vi "CleanHandler.init clean afg.vi"(0 "i ref in":refnum<vi>, 1 "CleanAfg":i32, 2 "amplitude [V]":dbl format="%.2f", 3 "ms timeout (100)":i32=100, 4 "frequency [Hz]":dbl format="%.2f", 5 "error in (no error)":errorcluster) -> (14 "i ref out":refnum<vi>, 17 "timed out":bool, 19 "error out":errorcluster)   [LabVIEW 2014, in "CleanHandler.lvlib"]
doc: "Sets the frequency [Hz] and amplitude [V] at the AFG with number CleanAFG. The numbering of the CleanAFGs starts with 0."
uses:
  CleanHandler.lvlib
  CS_Core/CSSystem/CoreDefs/CoreDefs.error_type.ctl
  CS_Core/CSSystem/CoreLib/CoreLib.double 2 byte array.vi
  CS_Core/CSSystem/CoreLib/CoreLib.lvlib
  CS_Core/BaseProcess/BaseProcess.lvlib
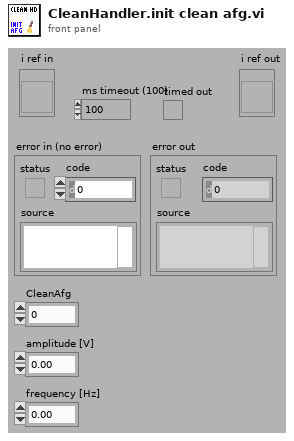
[diagram p1: front panel]
types:
  T1 = typedef "CoreDefs.error_type.ctl" = enum16{"no error", "can't load process", "can't unload process", "process does not exist", "can't install process", "can't remove process", "unknown function", "time out", "can't execute function", "duplicate queue name", "super not found", "caller queue invalid", "can't ping process", "unknown error", "VISA Error", "VISA timeout", "GPIB timeout", "GPIB error", "communication error", "data type mismatch", "can't read data from OPC server", "can't write data to OPC server", "OET error", "function not implemented", "process already exists", "invalid Shared Variable name", "error writing Shared Variable", "error reading Shared Variable", "invalid client name", "corrupt database", "unknown class", "call not authorized", "parameter out of range", "OET timeout: can't get data to modify", "invalid queue name", "requested operation incompatible with current state", "event undefined", "event disabled", "state undefined", "caller is not a friend", "EventBuilder: bad eventID", "EventBuilder: no DAQ devices", "a thread must not stop itself", "UNUSED ELEMENT4", "DiscArchiver: eventData incomplete", "DiscArchiver: eventData does not belong to run", "DiscArchiver: can't open file", "DiscArchiver: can't write to file", "DiscArchiver: available disc space low", "can't acquire semaphore", "error reading data from database", "notifier object is not existing", "can't register process", "can't unregister process", "illegal event type", "object disabled", "object already exists", "can't change state", "Instrument not found", "no connection to remote node", "invalid reference", "N/A", "UNUSED ELEMENT 1", "element not found", "illegal TCP/IP connection detected", "object does not exist", "invalid access ID", "unknown CS system", "invalid privilige", "unsupported data type", "unsupported server type", "IO server already exists", "Shared Variable already exists"}
  T2 = enum16{"simple", "synchronous", "asynchronous", "notification"}
  T3 = typedef "CoreDefs.rawDataType.ctl" = i8[]
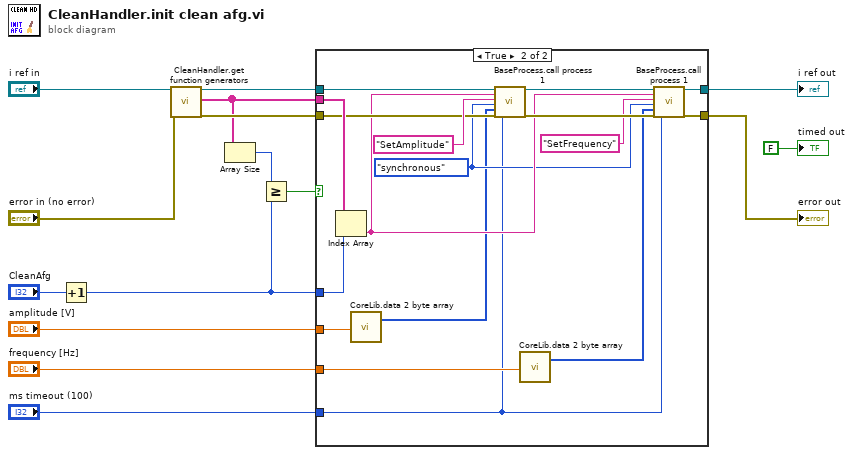
[diagram p0: block diagram]
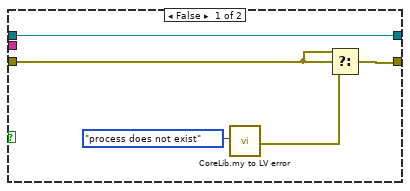
[diagram p2: hidden frame]
diagram:
  n1 = Increment(x="CleanAfg") -> (x+1=w5:i32)
  n2 = call "CleanHandler.get function generators.vi"("i ref in"="i ref in", "error in (no error)"="error in (no error)") -> ("i ref out"=w10:refnum<vi>, "function generators"=w6:string[], "error out"=w8:errorcluster)  [unwired: 14 in, 1 out]
  n3 = Array Size(array=w6) -> (size(s)=w12:i32)
  n4 = Greater Or Equal?(x=w12, y=w5) -> (x >= y?=w11:bool)
  n5 = case shown="True" w11 {
    tunnel: [w20 w31] -> w9
    tunnel: w10 -> [w20 w37]
    tunnel: w8 -> [w18 w33]
    tunnel: [w19 w30] -> w7
    tunnel: w6 -> [_ w36]
    tunnel: w5 -> [_ w35]
    tunnel: "amplitude [V]" -> [_ w32]
    tunnel: "frequency [Hz]" -> [_ w24]
    tunnel: "ms timeout (100)" -> [_ w23]
    frame False {
      n6 = call "CoreLib.my to LV error.vi"("ErrorTypes"=CoreDefs.error_type."process does not exist") -> ("myErrorCluster"=w17:errorcluster)  [unwired: 17 in, 1 out]
      n7 = Select(t=w18, s=w18, f=w17) -> (s? t:f=w19:errorcluster)
    }
    frame True {
      w25 = T2."synchronous" ("CallType")
      n8 = Index Array(array=w36, index=w35) -> (element=w27:string)
      n9 = call-poly "CoreLib.data 2 byte array.vi"("f64"=w32) -> ("byteArray out"=w21:T3)  [unwired: 18 in]
      n10 = call "BaseProcess.call process 1.vi"("i ref in"=w37, "Object"=w27, "Selector"="SetAmplitude", "CallType"=w25, "Data"=w21, "error in (no error)"=w33, "timeout (ms)"=w23) -> ("i ref out"=w29:refnum<vi>, "error out"=w28:errorcluster)  [unwired: 10 in, 1 out]
      n11 = call-poly "CoreLib.data 2 byte array.vi"("f64"=w24) -> ("byteArray out"=w22:T3)  [unwired: 18 in]
      n12 = call "BaseProcess.call process 1.vi"("i ref in"=w29, "Object"=w27, "Selector"="SetFrequency", "CallType"=w25, "Data"=w22, "error in (no error)"=w28, "timeout (ms)"=w23) -> ("i ref out"=w31:refnum<vi>, "error out"=w30:errorcluster)  [unwired: 10 in, 1 out]
    }
  }
  "error out" <- w7
  "i ref out" <- w9
  "timed out" <- FALSE ("timed out")
